vi "UHR-Fleezers Control (host) - Lorentz v3.vi"() -> ()   [LabVIEW 2014] (continued)
    n3456 = Bundle By Name(cluster=w4564, "Set 1"=w4563, "Set 2"=w4562) -> (w4334:cluster{"Set 1":dbl, "Set 2":dbl})
    n3457 = Divide(x=w4447, y=327.67) -> (x/y=→"Action (%)":dbl)
    n3458 = case shown="True" "Semi Passive Mode" {
      tunnel: w4313 -> [_ w4631]
      frame False {
      }
      frame True {
        n3459 = local read "Target Force (pN)"() -> (w4629:dbl)
        n3460 = Less?(x="Jump Force (pN)", y=w4629) -> (x < y?=w4627:bool)
        n3461 = case shown="False" w4627 {
          tunnel: "Jump Force (pN)" -> [w4637 w4640]
          tunnel: w4631 -> [w4636 w4639]
          tunnel: [w4635 w4638] -> w4630
          frame False {
            n3462 = Less?(x=w4637, y=w4636) -> (x < y?=w4635:bool)
          }
          frame True {
            n3463 = Greater?(x=w4640, y=w4639) -> (0:w4638:bool)
          }
        }
        n3464 = case shown="False" w4630 {
          frame False {
            n3465 = local read "Trap Pos. FB ON"() -> (w4632:bool)
            n3466 = case shown="False" w4632 {
              frame False {
              }
              frame True {
                n3467 = property on="Trap Pos. FB ON" class="Bool (strict)"("Val(Sgnl)"=FALSE) -> ()  [unwired: 2 in, 2 out]
              }
            }
          }
          frame True {
            n3468 = property on="Trap Pos. FB ON" class="Bool (strict)"("Val(Sgnl)"=TRUE) -> ()  [unwired: 2 in, 2 out]
          }
        }
      }
    }
    n3469 = local read "Trap X (AI1)"() -> (w4467:T15)
    n3470 = call "IR AOM word double to freq.vi"("Frequency Word In (double)"=w4405) -> ("Frequency Out (MHz)"=w4404:dbl)
    n3471 = call "IR AOM word double to freq.vi"("Frequency Word In (double)"=w4407) -> ("Frequency Out (MHz)"=w4406:dbl)
    n3472 = Divide(x=w4334, y=3276.7) -> (x/y=w4560:cluster{"Set 1":dbl, "Set 2":dbl})
    n3473 = Multiply(x=w4406, y=w4413) -> (x*y=w4412:dbl)
    "TTrig Sig (nm)" <- w4412
    n3474 = Multiply(x=w4404, y=w4413) -> (x*y=w4411:dbl)
    "TTrig Fin Thresh (nm)" <- w4411
    n3475 = local write "AI2 (V)"(w4560) -> ()
    n3476 = Bundle(cluster=w4467, "Trap 1"=w4454, "Trap 2"=w4453) -> (→"Trap X (AI1)":T15)
    n3477 = local read "Trap Pos. FB ON"() -> (w4320:bool)
    n3478 = local read "Dynamic Force FB (ronen)"() -> (w4321:bool)
    n3479 = Bundle(w4412, w4411) -> (→"TTrig":cluster{dbl, dbl})  [unwired: 1 in]
    n3480 = Compound Arithmetic op=AND(w4321, "Real time Offset file correction for setpoint", w4320) -> (w4322:bool)
    n3481 = case shown="True" w4322 {
      tunnel: w4332 -> [_ _]
      tunnel: w4318 -> [_ w4659]
      tunnel: w4315 -> [_ w4642]
      frame False {
      }
      frame True {
        # "Changed by Ronen - real time update of set point\naccording to offset file"
        n3482 = local read "T1 calibration"() -> (w4654:T9)
        n3483 = local read "Offset file step size"() -> (w4661:dbl)
        n3484 = local read "Setpoint offset\ncorrection values"() -> (w4658:dbl[])
        n3485 = Multiply(x="Target Force (pN)", y=2.0) -> (x*y=w4655:dbl)
        n3486 = local read "Negate Diff?"() -> (w4643:bool)
        n3487 = Unbundle By Name(w4654) -> ("T1 alpha_x (nm/V)"=w4653:dbl, "T1 kappa_x (pN/nm)"=w4652:dbl)
        n3488 = Divide(x=w4659, y=w4661) -> (x/y=w4662:dbl)
        n3489 = To Long Integer(number=w4662) -> (32bit integer=w4660:i32)
        n3490 = Index Array(array=w4658, index=w4660) -> (element=w4645:dbl)
        n3491 = Multiply(x=w4653, y=w4652) -> (x*y=w4651:dbl)
        n3492 = Select(t=1, s=w4643, f=-1) -> (s? t:f=w4646:i32)
        n3493 = Divide(x=w4655, y=w4651) -> (x/y=w4650:dbl)
        n3494 = Multiply(x=w4646, y=w4645) -> (x*y=w4644:dbl)
        n3495 = Add(x=w4650, y=w4644) -> (x+y=w4649:dbl)
        n3496 = To Fixed-Point(number=w4649) -> (fixed-point=w4641:fxp<+/-,16,1>)  [unwired: 1 in]
        "Actual Setpoint" <- w4641
        n3497 = xnode "Read/Write Control"("FPGA VI Reference In"=w4642, "Trap Pos. FB SP"=w4641) -> ()  [unwired: 1 in, 2 out]
      }
    }
    n3498 = local read "All FB On/Off"() -> (w4333:bool)
    n3499 = case shown="True" w4333 {
      tunnel: w4334 -> [_ w4665]
      frame False {
      }
      frame True {
        n3500 = Divide(x=w4665, y=3276.7) -> (x/y=w4663:cluster{"Set 1":dbl, "Set 2":dbl})
        n3501 = Unbundle By Name(w4663) -> ("Set 1"=w4670:dbl, "Set 2"=w4669:dbl)
        n3502 = Greater?(x=w4670, y="Feedback Auto-Off threshold") -> (0:w4668:bool)
        n3503 = Greater?(x=w4669, y="Feedback Auto-Off threshold") -> (0:w4667:bool)
        n3504 = Or(x=w4668, y=w4667) -> (x .or. y?=w4666:bool)
        n3505 = case shown="True" w4666 {
          frame False {
          }
          frame True {
            n3506 = property on="All FB On/Off" class="Bool (strict)"("Val(Sgnl)"=FALSE) -> ()  [unwired: 2 in, 2 out]
          }
        }
      }
    }
    n3507 = flat-sequence "To save data" {
      tunnel: [w5368] -> w4583
      tunnel: [w5369] -> w4582
      tunnel: w4545 -> [w5362]
      tunnel: w4256 -> [w5366]
      tunnel: ["Save Calibration"] -> w4557
      tunnel: w4304 -> [w5365]
      tunnel: [w5358] -> w4554
      tunnel: [w5355] -> w4553
      tunnel: [w5352] -> w4552
      tunnel: w4544 -> [w5354]
      tunnel: w4283 -> [w5348]
      tunnel: [w5348] -> w4508
      tunnel: ["Start Saving"] -> w4488
      tunnel: [w5343] -> w4437
      tunnel: [w5342] -> w4436
      tunnel: [w5339] -> w4338
      tunnel: [w5335] -> w4326
      tunnel: w4583 -> [w5680]
      tunnel: w4582 -> [w5679]
      tunnel: w4305 -> [w5678]
      tunnel: w4557 -> [w5677]
      tunnel: w4554 -> [w5675]
      tunnel: w4553 -> [w5674]
      tunnel: w4552 -> [w5673]
      tunnel: w4279 -> [w5672]
      tunnel: w4300 -> [w5671]
      tunnel: w4508 -> [w5670]
      tunnel: w4488 -> [w5669]
      tunnel: w4345 -> [w5668]
      tunnel: w4387 -> [w5667]
      tunnel: w4437 -> [w5666]
      tunnel: w4436 -> [w5665]
      tunnel: w4435 -> [w5664]
      tunnel: w4228 -> [w5663]
      tunnel: w4294 -> [w5662]
      tunnel: w4338 -> [w5661]
      tunnel: w4326 -> [w5660]
      frame #0 {
        # "Changed by Ronen - we don't have a database so we disabled this"
        n3508 = Or(x="Save N Sets", y="Start Saving") -> (x .or. y?=w5349:bool)
        n3509 = To Double Precision Float(number=w5365) -> (double precision float=w5359:dbl)
        n3510 = Build Array(w5349, "Save Calibration", w5362, w5354, "Flow Cal") -> (w5364:bool[])
        n3511 = Compound Arithmetic op=OR("Save Calibration", w5362, w5349, w5354, "Flow Cal") -> (w5367:bool)
        n3512 = Boolean Array To Number(Boolean array=w5364) -> (number=w5361:u32)
        n3513 = feedback #21(FALSE ("Save APD Data\nwith Trap Data")) -> (w5344:bool)
        n3514 = feedback #22(refnum<k0> refnum) -> (w5370:refnum<file>)
        n3515 = feedback #23(FALSE ("Save APD Data\nwith Trap Data")) -> (w5353:bool)
        n3516 = feedback #24(0) -> (w5372:i32)
        n3517 = feedback #25() -> (w5360:u32)  [unwired: 1 out]
        n3518 = feedback #26(refnum<k0> refnum) -> (w5340:refnum<file>)
        n3519 = feedback #27(refnum<k0> refnum) -> (w5346:refnum<file>)
        n3520 = feedback #28(refnum<k0> refnum) -> (w5336:refnum<file>)
        n3521 = feedback #29(refnum<k0> refnum) -> (w5356:refnum<file>)
        n3522 = case shown="True" w5367 {
          tunnel: [w5381 1] -> w5368
          tunnel: w5372 -> [w5383 _]
          tunnel: [w5382 w5415] -> w5369
          tunnel: w5370 -> [w5382 _]
          tunnel: w5366 -> [_ w5433]
          tunnel: w5359 -> [_ w5431]
          tunnel: w5361 -> [_ w5434]
          tunnel: [w5380 w5414] -> w5358
          tunnel: w5360 -> [w5380 _]
          tunnel: [w5379 w5412] -> w5355
          tunnel: w5356 -> [w5379 _]
          tunnel: [w5378 w5411] -> w5352
          tunnel: w5353 -> [w5378 _]
          tunnel: "Start Saving" -> [_ w5409]
          tunnel: w5348 -> [_ w5408]
          tunnel: [w5377 w5401] -> w5342
          tunnel: w5346 -> [w5377 _]
          tunnel: [w5376 w5400] -> w5343
          tunnel: w5344 -> [w5376 _]
          tunnel: [w5375 w5386] -> w5339
          tunnel: w5340 -> [w5375 _]
          tunnel: [w5374 w5384] -> w5335
          tunnel: w5336 -> [w5374 _]
          frame False {
            n3523 = Increment(x=w5383) -> (x+1=w5381:i32)
          }
          frame True {
            w5385 = FALSE ("Start Saving")
            w5410 = 10.0  # File Version
            w5417 = FALSE ("prepend array or string size? (T)")
            w5416 = T45."big-endian, network order" ("byte order (0:big-endian, network order)")
            # "Ronen Changed the create file - changed data folder to c:\\Data"
            # "Save trap position\ndata"
            n3524 = Array Size(array=w5408) -> (size(s)=w5407:i32)
            n3525 = To Double Precision Float(number=w5407) -> (double precision float=w5406:dbl)
            n3526 = local read "BD 1 Frequency 1 (MHz)"() -> (w5430:dbl)
            n3527 = local read "BD 2 Frequency 1 (MHz)"() -> (w5429:dbl)
            n3528 = local read "BD 1 Frequency 2 (MHz)"() -> (w5428:dbl)
            n3529 = local read "BD 2 Frequency 2 (MHz)"() -> (w5427:dbl)
            n3530 = local read "BD 1 Frequency 3 (MHz)"() -> (w5426:dbl)
            n3531 = local read "BD 2 Frequency 3 (MHz)"() -> (w5425:dbl)
            n3532 = local write "Flow Cal"(w5385) -> ()
            n3533 = local write "Save Calibration"(w5385) -> ()
            n3534 = local write "Start Saving"(w5385) -> ()
            n3535 = Build Array("Save APD Data\nwith Trap Data", "Save Trap Pos. Data") -> (w5403:bool[])
            n3536 = Boolean Array To Number(Boolean array=w5403) -> (number=w5402:u32)
            n3537 = Build Array(w5430, w5429, w5428, w5427, w5426, w5425) -> (w5424:dbl[])
            n3538 = case shown="16" w5434 {
              tunnel: w5433 -> [w5534 w5561 w5577 w5615 w5652]
              tunnel: w5406 -> [w5539 w5568 w5597 w5634 w5657]
              tunnel: w5431 -> [w5538 w5567 w5596 w5633 w5656]
              tunnel: [w5535 w5563 w5588 w5625 w5653] -> w5422
              tunnel: [w5526 "Cal sets to save" w5578 w5616 w5639] -> w5414
              tunnel: w5424 -> [w5536 w5564 w5590 w5627 w5654]
              tunnel: "Save APD Data\nwith Trap Data" -> [w5533 w5550 w5574 w5613 w5651]
              tunnel: [w5533 w5548 w5574 w5613 w5651] -> w5411
              tunnel: w5410 -> [w5529 w5557 w5572 w5611 w5647]
              tunnel: w5409 -> [w5528 _ _ _ _]
              tunnel: [w5519 w5556 w5571 w5601 w5646] -> w5400
              tunnel: "Save Trap Pos. Data" -> [w5519 w5555 w5571 w5601 w5646]
              tunnel: w5402 -> [w5518 w5554 w5570 w5600 w5645]
              frame 1, Default {
                # "timeseries"
                n3539 = case shown="True" "Profile" {
                  tunnel: [w5542 w5546] -> w5523
                  tunnel: [w5542 w5545] -> w5522
                  tunnel: [w5542 w5544] -> w5521
                  tunnel: [w5542 w5543] -> w5520
                  frame False {
                    w5542 = 0.0 ("f")
                  }
                  frame True {
                    n3540 = local read "Current Position"() -> (w5547:cluster{dbl, dbl, dbl})
                    n3541 = local read "Y change (mm)"() -> (w5543:dbl)
                    n3542 = Unbundle(w5547) -> (w5546:dbl, w5545:dbl, w5544:dbl)
                  }
                }
                n3543 = local read "Save ave N"() -> (w5541:dbl)
                n3544 = Multiply(x=w5541, y=w5534) -> (x*y=w5540:dbl)
                n3545 = To Double Precision Float(number=w5518) -> (double precision float=w5532:dbl)
                n3546 = Build Array(w5529, w5534, w5540, w5539, w5538, 0.0 ("f")) -> (w5537:dbl[])
                n3547 = Build Array(w5532, w5523, w5522, w5521, w5520) -> (w5530:dbl[])
                n3548 = Select(t=u32 4000000000, s=w5528, f="N sets to save") -> (s? t:f=w5526:u32)
                n3549 = Build Array (concatenate)(w5537, w5536, w5530) -> (w5535:dbl[])
              }
              frame 2 {
                w5559 = 0.0 ("f")
                w5549 = FALSE ("Save APD Data\nwith Trap Data")
                # "For diagnostics save trap position\ndata during cal"
                # "calibration"
                n3550 = Boolean To (0,1)(Boolean=w5549) -> (0, 1=w5553:i16)
                n3551 = Select(t=w5550, s="Save trap pos with cal", f=w5549) -> (s? t:f=w5548:bool)
                n3552 = Select(t=w5555, s="Save trap pos with cal", f=w5549) -> (s? t:f=w5556:bool)
                n3553 = Select(t=w5554, s="Save trap pos with cal", f=w5553) -> (s? t:f=w5552:u32)
                n3554 = To Double Precision Float(number=w5552) -> (double precision float=w5560:dbl)
                n3555 = Build Array(w5557, w5561, w5561, w5568, w5567, 1.0 ("t")) -> (w5565:dbl[])
                n3556 = Build Array(w5560, w5559, w5559, w5559, w5559) -> (w5558:dbl[])
                n3557 = Build Array (concatenate)(w5565, w5564, w5558) -> (w5563:dbl[])
                "Calibrating Trap..." <- TRUE ("Calibrating...")
              }
              frame 4 {
                w5575 = 0.0 ("f")
                # "scan dir (x/y = 0/1)"
                # "cycles/step"
                # "n scans (f/b)"
                # "steps"
                # "freq. range"
                # "AOD raster scan"
                n3558 = local read "Number of F/B Scans (AOD)"() -> (w5582:u16)
                n3559 = local read "Cycles/step (AOD)"() -> (w5584:u64)
                n3560 = local read "Scan Range (MHz)"() -> (w5587:dbl)
                n3561 = local read "Scan steps (AOD)"() -> (w5586:u64)
                n3562 = local read "Scan BD"() -> (w5594:bool)
                n3563 = local read "Save ave N"() -> (w5599:dbl)
                n3564 = Boolean To (0,1)(Boolean=w5594) -> (0, 1=w5593:i16)
                n3565 = To Double Precision Float(number=w5582) -> (double precision float=w5581:dbl)
                n3566 = To Double Precision Float(number=w5586) -> (double precision float=w5585:dbl)
                n3567 = To Double Precision Float(number=w5584) -> (double precision float=w5583:dbl)
                n3568 = To Double Precision Float(number=w5593) -> (double precision float=w5592:dbl)
                n3569 = Multiply(x=w5599, y=w5577) -> (x*y=w5598:dbl)
                n3570 = To Double Precision Float(number=w5570) -> (double precision float=w5576:dbl)
                n3571 = Build Array(w5576, w5575, w5575, w5575, w5575) -> (w5573:dbl[])
                n3572 = local read "N sets should be saved"() -> (w5579:dbl)
                n3573 = Build Array(w5592, w5587, w5585, w5583, w5581) -> (w5589:dbl[])
                n3574 = Build Array(w5572, w5577, w5598, w5597, w5596, 2.0 ("t")) -> (w5591:dbl[])
                n3575 = Round Toward +Infinity(x=w5579) -> (ceil(x): smallest int >= x=w5580:dbl)
                n3576 = Build Array (concatenate)(w5591, w5590, w5573, w5589) -> (w5588:dbl[])
                n3577 = To Unsigned Long Integer(number=w5580) -> (unsigned 32bit integer=w5578:u32)
              }
              frame 8 {
                w5608 = 0.0 ("f")
                # "MCL raster scan"
                n3578 = local read "Number of scans (MCL)"() -> (w5603:u64)
                n3579 = local read "2D or 1D Scan"() -> (w5605:bool)
                n3580 = local read "Scan lines (y)"() -> (w5602:u64)
                n3581 = local read "Scan Range (V)\n(of steps)"() -> (w5624:dbl)
                n3582 = local read "Fast Scan Dir"() -> (w5631:bool)
                n3583 = local read "Cycles/step (MCL)"() -> (w5621:u64)
                n3584 = local read "Scan steps (MCL)"() -> (w5623:u64)
                n3585 = Select(t=w5602, s=w5605, f=w5603) -> (s? t:f=w5604:u64)
                n3586 = Boolean To (0,1)(Boolean=w5605) -> (0, 1=w5607:i16)
                n3587 = local read "Save ave N"() -> (w5636:dbl)
                n3588 = local read "Initial X"() -> (w5610:dbl)
                n3589 = local read "Initial Y"() -> (w5609:dbl)
                n3590 = To Double Precision Float(number=w5607) -> (double precision float=w5606:dbl)
                n3591 = Boolean To (0,1)(Boolean=w5631) -> (0, 1=w5630:i16)
                n3592 = To Double Precision Float(number=w5604) -> (double precision float=w5619:dbl)
                n3593 = To Double Precision Float(number=w5623) -> (double precision float=w5622:dbl)
                n3594 = To Double Precision Float(number=w5621) -> (double precision float=w5620:dbl)
                n3595 = To Double Precision Float(number=w5630) -> (double precision float=w5629:dbl)
                n3596 = Multiply(x=w5636, y=w5615) -> (x*y=w5635:dbl)
                n3597 = To Double Precision Float(number=w5600) -> (double precision float=w5614:dbl)
                n3598 = local read "N sets should be saved (MCL)"() -> (w5617:dbl)
                n3599 = Build Array(w5614, w5606, w5608, w5608, w5608) -> (w5612:dbl[])
                n3600 = Build Array(w5629, w5624, w5622, w5620, w5619, w5610, w5609) -> (w5626:dbl[])
                n3601 = Build Array(w5611, w5615, w5635, w5634, w5633, 3.0 ("t")) -> (w5628:dbl[])
                n3602 = Round Toward +Infinity(x=w5617) -> (ceil(x): smallest int >= x=w5618:dbl)
                n3603 = Build Array (concatenate)(w5628, w5627, w5612, w5626) -> (w5625:dbl[])
                n3604 = To Unsigned Long Integer(number=w5618) -> (unsigned 32bit integer=w5616:u32)
              }
              frame 16 {
                w5638 = 0.0
                # "Flow calibration - added by Ronen: Number\nof saved sets is distance (1 mm) divided by \nspeed +1.5 spare second divided by the time of\nset measurement, 0.2 sec for 2 set interlace"
                # "timeseries"
                n3605 = local read "Save ave N"() -> (w5659:dbl)
                n3606 = Reciprocal(x=0.0) -> (1/x=w5644:dbl)
                n3607 = Add(x=w5644, y=1.5) -> (x+y=w5642:dbl)
                n3608 = Multiply(x=w5659, y=w5652) -> (x*y=w5658:dbl)
                n3609 = Divide(x=w5642, y=0.2) -> (x/y=w5640:dbl)
                n3610 = To Double Precision Float(number=w5645) -> (double precision float=w5650:dbl)
                n3611 = To Unsigned Long Integer(number=w5640) -> (unsigned 32bit integer=w5639:u32)
                n3612 = Build Array(w5647, w5652, w5658, w5657, w5656, 4.0 ("f")) -> (w5655:dbl[])
                n3613 = Build Array(w5650, w5638, w5638, w5638, w5638) -> (w5648:dbl[])
                n3614 = Build Array (concatenate)(w5655, w5654, w5648) -> (w5653:dbl[])
              }
            }
            n3615 = local read "Index"() -> (w5439:dbl)
            n3616 = call "Create new save file.vi"("Insert"="", "Ext"=".dat", "Index In"=w5439) -> ("Path Out"=w5388:path, "Index Out"=w5413:dbl)
            n3617 = local write "Save file name"(w5388) -> ()
            n3618 = local write "Index"(w5413) -> ()
            n3619 = local write "Save index"(w5413) -> ()
            n3620 = case shown="True" "Save Event Log?" {
              tunnel: w5388 -> [_ w5453]
              tunnel: [refnum<k0> refnum w5452] -> w5386
              frame False {
              }
              frame True {
                (unwired) FALSE ("prepend array or string size? (T)")
                n3621 = Path To String(path=w5453) -> (string=w5464:string)
                n3622 = String Length(string=w5464) -> (length=w5463:i32)
                n3623 = Subtract(x=w5463, y=4) -> (x-y=w5461:i32)
                n3624 = String Subset(string=w5464, length (rest)=w5461) -> (substring=w5460:string)  [unwired: 1 out]
                n3625 = Concatenate Strings(w5460, "_log.txt" ("string")) -> (w5458:string)
                n3626 = String To Path(string=w5458) -> (path=w5454:path)
                n3627 = Open/Create/Replace File(file path (use dialog)=w5454, operation (0:open)=T44."create", access (0:read/write)=enum16{"read/write", "read-only", "write-only"}."write-only") -> (refnum out=w5455:refnum<file>)  [unwired: 1 in, 4 out]
                n3628 = Deny Access(7:w5455) -> (3:w5452:refnum<file>)  [unwired: 1 in, 2 out]
                n3629 = call "write to event log.vi"("log file ref"=w5452, "time"=0.0, "input string"="start log") -> ()  [unwired: 8 in]
              }
            }
            "log file ref" <- w5386
            n3630 = Array Size(array=w5422) -> (size(s)=w5423:i32)
            n3631 = Open/Create/Replace File(file path (use dialog)=w5388, operation (0:open)=T44."create", access (0:read/write)=enum16{"read/write", "read-only", "write-only"}."write-only") -> (refnum out=w5436:refnum<file>)  [unwired: 1 in, 4 out]
            n3632 = local write "Saving..."(TRUE ("Saving...")) -> ()
            n3633 = To Double Precision Float(number=w5423) -> (double precision float=w5421:dbl)
            n3634 = String Length(string="Comment (data description)") -> (length=w5420:i32)
            n3635 = To Double Precision Float(number=w5420) -> (double precision float=w5419:dbl)
            n3636 = Deny Access(7:w5436) -> (3:w5435:refnum<file>)  [unwired: 1 in, 2 out]
            n3637 = Build Array (concatenate)(w5421, w5422, w5419) -> (w5398:dbl[])
            n3638 = case "If fluorescence data to be saved" shown="True" w5411 {
              tunnel: w5388 -> [_ w5517]
              tunnel: [w5487 w5500] -> w5412
              tunnel: [w5487 w5488] -> w5384
              frame False {
                w5487 = refnum<k0> refnum
              }
              frame True {
                w5499 = 0.0
                w5492 = T44."create" ("operation (0:open)")
                w5493 = enum16{"read/write", "read-only", "write-only"}."write-only" ("access (0:read/write)")
                n3639 = local read "APD Integration Time (s)"() -> (w5505:dbl)
                n3640 = local read "N APD Samp/step"() -> (w5498:dbl)
                n3641 = local read "Number of APDs"() -> (w5497:u8)
                n3642 = Path To String(path=w5517) -> (string=w5516:string)
                n3643 = String Length(string=w5516) -> (length=w5515:i32)
                n3644 = Subtract(x=w5515, y=4) -> (x-y=w5513:i32)
                n3645 = String Subset(string=w5516, length (rest)=w5513) -> (substring=w5496:string)  [unwired: 1 out]
                n3646 = Build Array(w5505, w5498, w5497, w5499, w5499, w5499, w5499, w5499) -> (w5502:dbl[])
                n3647 = Concatenate Strings(w5496, "_green.dat") -> (w5494:string)
                n3648 = Concatenate Strings(w5496, "_fl.dat" ("string")) -> (w5511:string)
                n3649 = Array Size(array=w5502) -> (size(s)=w5504:i32)
                n3650 = String To Path(string=w5511) -> (path=w5509:path)
                n3651 = Open/Create/Replace File(file path (use dialog)=w5509, operation (0:open)=w5492, access (0:read/write)=w5493) -> (refnum out=w5510:refnum<file>)  [unwired: 1 in, 4 out]
                n3652 = Deny Access(7:w5510) -> (3:w5506:refnum<file>)  [unwired: 1 in, 2 out]
                n3653 = String To Path(string=w5494) -> (path=w5491:path)
                n3654 = To Double Precision Float(number=w5504) -> (double precision float=w5503:dbl)
                n3655 = Build Array (concatenate)(w5503, w5502) -> (w5501:dbl[])
                n3656 = Write to Binary File(file (use dialog)=w5506, data=w5501, 5:FALSE ("prepend array or string size? (T)"), 9:T45."big-endian, network order" ("byte order (0:big-endian, network order)")) -> (refnum out=w5500:refnum<file>)  [unwired: 1 in, 3 out]
                n3657 = Open/Create/Replace File(file path (use dialog)=w5491, operation (0:open)=w5492, access (0:read/write)=w5493) -> (refnum out=w5489:refnum<file>, error out=w5490:errorcluster)  [unwired: 3 in, 1 out]
                n3658 = Deny Access(4:w5490, 7:w5489) -> (3:w5488:refnum<file>)  [unwired: 1 in, 1 out]
              }
            }
            n3659 = case shown="True" w5400 {
              tunnel: w5388 -> [_ w5472]
              tunnel: [refnum<k0> refnum w5471] -> w5401
              frame False {
              }
              frame True {
                w5467 = 0.0 ("element")
                n3660 = Path To String(path=w5472) -> (string=w5486:string)
                n3661 = Build Array(w5467, w5467, w5467, w5467, w5467, w5467, w5467, w5467) -> (w5468:dbl[])
                n3662 = String Length(string=w5486) -> (length=w5485:i32)
                n3663 = Subtract(x=w5485, y=4) -> (x-y=w5483:i32)
                n3664 = Array Size(array=w5468) -> (size(s)=w5470:i32)
                n3665 = String Subset(string=w5486, length (rest)=w5483) -> (substring=w5482:string)  [unwired: 1 out]
                n3666 = To Double Precision Float(number=w5470) -> (double precision float=w5469:dbl)
                n3667 = Concatenate Strings(w5482, "_pos.dat" ("string")) -> (w5480:string)
                n3668 = Build Array (concatenate)(w5469, w5468) -> (w5466:dbl[])
                n3669 = String To Path(string=w5480) -> (path=w5476:path)
                n3670 = Open/Create/Replace File(file path (use dialog)=w5476, operation (0:open)=T44."create", access (0:read/write)=enum16{"read/write", "read-only", "write-only"}."write-only") -> (refnum out=w5477:refnum<file>)  [unwired: 1 in, 4 out]
                n3671 = Deny Access(7:w5477) -> (3:w5473:refnum<file>)  [unwired: 1 in, 2 out]
                n3672 = Write to Binary File(file (use dialog)=w5473, data=w5466, 5:FALSE ("prepend array or string size? (T)"), 9:T45."big-endian, network order" ("byte order (0:big-endian, network order)")) -> (refnum out=w5471:refnum<file>)  [unwired: 1 in, 3 out]
              }
            }
            n3673 = Write to Binary File(file (use dialog)=w5435, data=w5398, 5:w5417, 9:w5416) -> (refnum out=w5418:refnum<file>)  [unwired: 1 in, 3 out]
            n3674 = Write to Binary File(file (use dialog)=w5418, data="Comment (data description)", 5:w5417, 9:w5416) -> (refnum out=w5415:refnum<file>)  [unwired: 1 in, 3 out]
            n3675 = local read "connection reference"() -> (w5399:T25)
            n3676 = Bundle("Comment (data description)"="Comment (data description)", "Channel 1 Buffer"="Channel 1 Buffer", "Channel 2 Buffer"="Channel 2 Buffer", "Channel 3 Buffer"="Channel 3 Buffer", "Title"="Title", "DNA Construct"="DNA Construct", "Bead diameter"="Bead diameter", "Name"="Name") -> (w5389:T64)  [unwired: 1 in]
            n3677 = disable-structure shown="Disabled" {
              disable-tunnel: w5399 -> [w5447 _]
              disable-tunnel: w5398 -> [w5445 _]
              disable-tunnel: w5389 -> [w5444 _]
              disable-tunnel: w5388 -> [w5443 _]
              frame Disabled {
                n3678 = call "MattFileCreator-v9.vi"("Comments"=w5444, "Input Array"=w5445, "File path"=w5443, "table"="labview", "connection reference"=w5447) -> ("connection reference out"=w5446:T25)  [unwired: 5 in, 1 out]
                n3679 = local write "connection reference"(w5446) -> ()
              }
              frame Enabled {
              }
            }
          }
        }
        n3680 = feedback-in #21(w5343) -> ()
        n3681 = feedback-in #22(w5369) -> ()
        n3682 = feedback-in #23(w5352) -> ()
        n3683 = feedback-in #24(w5368) -> ()
        n3684 = feedback-in #25(w5358) -> ()
        n3685 = feedback-in #26(w5339) -> ()
        n3686 = feedback-in #27(w5342) -> ()
        n3687 = feedback-in #28(w5335) -> ()
        n3688 = feedback-in #29(w5355) -> ()
      }
      frame #1 {
        n3689 = local read "Saving..."() -> (w5676:bool)
        n3690 = case shown="True" w5676 {
          tunnel: w5680 -> [_ w5694]
          tunnel: w5679 -> [_ w5708]
          tunnel: w5678 -> [_ w5704]
          tunnel: w5677 -> [_ w5703]
          tunnel: w5675 -> [_ w5702]
          tunnel: w5674 -> [_ w5697]
          tunnel: w5673 -> [_ w5696]
          tunnel: w5672 -> [_ w5695]
          tunnel: w5671 -> [_ w5693]
          tunnel: w5670 -> [_ w5691]
          tunnel: w5669 -> [_ w5690]
          tunnel: w5668 -> [_ w5689]
          tunnel: w5667 -> [_ w5688]
          tunnel: w5666 -> [_ w5687]
          tunnel: w5665 -> [_ w5686]
          tunnel: w5664 -> [_ w5685]
          tunnel: w5663 -> [_ w5684]
          tunnel: w5662 -> [_ w5683]
          tunnel: w5661 -> [_ w5682]
          tunnel: w5660 -> [_ w5681]
          frame False {
          }
          frame True {
            n3691 = Multiply(x=w5694, y=w5693) -> (x*y=→"Time (s)":dbl)
            n3692 = Less Or Equal?(x=w5694, y=w5702) -> (x <= y?=w5706:bool)
            n3693 = Compound Arithmetic op=OR("Stop Saving", "Abort save 2") -> (w5698:bool)
            n3694 = Not(x=w5698) -> (.not. x?=w5707:bool)
            n3695 = And(x=w5706, y=w5707) -> (x .and. y?=w5705:bool)
            n3696 = case shown="True" w5705 {
              tunnel: w5708 -> [w5718 w5819]
              tunnel: [0.0 w5822] -> w5701
              tunnel: w5694 -> [_ w5820]
              tunnel: w5702 -> [_ w5821]
              tunnel: w5704 -> [_ w5816]
              tunnel: w5703 -> [_ _]
              tunnel: w5697 -> [w5716 w5809]
              tunnel: w5696 -> [w5715 w5810]
              tunnel: w5695 -> [_ w5808]
              tunnel: w5691 -> [_ w5807]
              tunnel: w5690 -> [_ w5725]
              tunnel: w5689 -> [_ w5800]
              tunnel: w5688 -> [_ w5747]
              tunnel: w5687 -> [w5712 w5764]
              tunnel: w5686 -> [w5713 w5763]
              tunnel: w5685 -> [_ w5760]
              tunnel: w5684 -> [_ w5758]
              tunnel: w5683 -> [_ w5724]
              tunnel: w5682 -> [w5711 _]
              tunnel: w5681 -> [w5709 w5723]
              frame False {
                w5714 = FALSE
                n3697 = Close File(refnum=w5718) -> ()  [unwired: 1 in, 2 out]
                n3698 = case shown="True" w5715 {
                  tunnel: w5716 -> [_ w5722]
                  tunnel: w5709 -> [_ w5721]
                  frame False {
                  }
                  frame True {
                    n3699 = Close File(refnum=w5722) -> ()  [unwired: 1 in, 2 out]
                    n3700 = Close File(refnum=w5721) -> ()  [unwired: 1 in, 2 out]
                  }
                }
                n3701 = case shown="True" w5712 {
                  tunnel: w5713 -> [_ w5720]
                  frame False {
                  }
                  frame True {
                    n3702 = Close File(refnum=w5720) -> ()  [unwired: 1 in, 2 out]
                  }
                }
                n3703 = local read "Save Event Log?"() -> (w5710:bool)
                n3704 = case shown="True" w5710 {
                  tunnel: w5711 -> [_ w5719]
                  frame False {
                  }
                  frame True {
                    n3705 = Close File(refnum=w5719) -> ()  [unwired: 1 in, 2 out]
                  }
                }
                n3706 = local write "Raster Scanning..."(w5714) -> ()
                n3707 = local write "Calibrating Trap..."(w5714) -> ()
                n3708 = call <vilib>:"Beep.vi"() -> ()  [unwired: 3 in, 9 out]
                n3709 = local write "Stop Saving"(w5714) -> ()
                "Saving..." <- w5714
              }
              frame True {
                n3710 = local read "Calibrating Trap..."() -> (w5811:bool)
                n3711 = case "Write fl. data" shown="True" w5810 {
                  tunnel: w5809 -> [_ w5852]
                  tunnel: w5808 -> [_ w5851]
                  tunnel: w5723 -> [_ w5845]
                  frame False {
                  }
                  frame True {
                    w5844 = FALSE ("prepend array or string size? (T)")
                    w5846 = T45."big-endian, network order" ("byte order (0:big-endian, network order)")
                    n3712 = property on="Green Laser ON" class="Bool (strict)"() -> ("Value"=w5850:bool)  [unwired: 2 in, 2 out]
                    n3713 = property on="Green Intensity % (FB OFF)" class="DigNum (strict)"() -> ("Value"=w5849:dbl)  [unwired: 2 in, 2 out]
                    n3714 = Boolean To (0,1)(Boolean=w5850) -> (0, 1=w5848:i16)
                    n3715 = Multiply(x=w5848, y=w5849) -> (x*y=w5847:dbl)
                    n3716 = Write to Binary File(file (use dialog)=w5852, data=w5851, 5:w5844, 9:w5846) -> ()  [unwired: 1 in, 4 out]
                    n3717 = Write to Binary File(file (use dialog)=w5845, data=w5847, 5:w5844, 9:w5846) -> ()  [unwired: 2 in, 3 out]
                  }
                }
                n3718 = Greater?(x="Save ave N", y=1.0) -> (0:w5814:bool)
                n3719 = Not(x=w5811) -> (.not. x?=w5813:bool)
                n3720 = And(x=w5813, y=w5814) -> (x .and. y?=w5761:bool)
                n3721 = case shown="True" w5761 {
                  tunnel: w5760 -> [w5825 w5836]
                  tunnel: [w5825 w5828] -> w5759
                  tunnel: "Save ave N" -> [_ w5829]
                  frame False {
                  }
                  frame True {
                    w5826 = 2 ("dimension size")
                    n3722 = Array Size(array=w5836) -> (size(s)=w5830:i32)
                    n3723 = Divide(x=w5830, y=w5826) -> (x/y=w5834:dbl)
                    n3724 = Reshape Array(w5836, w5834, w5826) -> (w5835:u64[][])
                    n3725 = Transpose 2D Array(2D array=w5835) -> (transposed array=w5833:u64[][])
                    n3726 = for {
                      tunnel: w5833 -> [w5838] mode=indexing
                      tunnel: [w5837] -> w5827 mode=indexing
                      tunnel: w5829 -> [w5839]
                      workers-P: _ -> [_]
                      n3727 = call "downsample 1D array - U64.vi"("Ave N"=w5839, "Array In"=w5838) -> ("Array Out"=w5837:u64[])  [unwired: 1 in]
                    }
                    n3728 = Transpose 2D Array(2D array=w5827) -> (transposed array=w5832:u64[][])
                    n3729 = Divide(x=w5830, y=w5829) -> (x/y=w5831:dbl)
                    n3730 = Reshape Array(w5832, w5831) -> (w5828:u64[])
                  }
                }
                n3731 = case shown="True" w5761 {
                  tunnel: w5816 -> [w5853 w5865]
                  tunnel: [w5853 w5857] -> w5812
                  tunnel: "Save ave N" -> [_ w5858]
                  tunnel: w5807 -> [_ w5856]
                  frame False {
                  }
                  frame True {
                    n3732 = Array Size(array=w5865) -> (size(s)=w5859:i32)
                    n3733 = Array Size(array=w5856) -> (size(s)=w5855:i32)
                    n3734 = Divide(x=w5859, y=w5855) -> (x/y=w5863:dbl)
                    n3735 = Reshape Array(w5865, w5863, w5855) -> (w5864:i16[][])
                    n3736 = Transpose 2D Array(2D array=w5864) -> (transposed array=w5862:i16[][])
                    n3737 = for {
                      tunnel: w5862 -> [w5868] mode=indexing
                      tunnel: [w5867] -> w5854 mode=indexing
                      tunnel: w5858 -> [w5866]
                      workers-P: _ -> [_]
                      n3738 = call "downsample 1D array - I16 to F32.vi"("Ave N"=w5866, "Array In"=w5868) -> ("Array Out"=w5867:sgl[])  [unwired: 1 in]
                    }
                    n3739 = Transpose 2D Array(2D array=w5854) -> (transposed array=w5861:sgl[][])
                    n3740 = Divide(x=w5859, y=w5858) -> (x/y=w5860:dbl)
                    n3741 = Reshape Array(w5861, w5860) -> (w5857:sgl[])
                  }
                }
                n3742 = Index Array(array=w5747, index=2) -> (element=w5748:waveform(dbl))
                n3743 = Index Array(array=w5747, index=1) -> (element=w5781:waveform(dbl))
                n3744 = Index Array(array=w5747, index=0) -> (element=w5783:waveform(dbl))
                n3745 = Unbundle By Name(w5748) -> ("Y"=w5750:dbl[])
                n3746 = Unbundle By Name(w5781) -> ("Y"=w5785:dbl[])
                n3747 = Unbundle By Name(w5783) -> ("Y"=w5793:dbl[])
                n3748 = case "Write trap pos. data" shown="True" w5764 {
                  tunnel: w5763 -> [_ w5841]
                  tunnel: w5759 -> [_ w5840]
                  frame False {
                  }
                  frame True {
                    n3749 = Write to Binary File(file (use dialog)=w5841, data=w5840, 5:FALSE ("prepend array or string size? (T)"), 9:T45."big-endian, network order" ("byte order (0:big-endian, network order)")) -> ()  [unwired: 1 in, 4 out]
                  }
                }
                n3750 = Write to Binary File(file (use dialog)=w5819, data=w5812, 5:FALSE ("prepend array or string size? (T)"), 9:T45."big-endian, network order" ("byte order (0:big-endian, network order)")) -> ()  [unwired: 1 in, 4 out]
                n3751 = feedback #30(w5750) -> (w5751:dbl[])
                n3752 = Build Array (concatenate)(w5751, w5750) -> (w5746:dbl[])
                n3753 = Select(t=w5750, s=w5725, f=w5746) -> (s? t:f=w5736:dbl[])
                n3754 = feedback-in #30(w5736) -> ()
                n3755 = feedback #31(w5785) -> (w5787:dbl[])
                n3756 = Build Array (concatenate)(w5787, w5785) -> (w5786:dbl[])
                n3757 = Select(t=w5785, s=w5725, f=w5786) -> (s? t:f=w5775:dbl[])
                n3758 = feedback-in #31(w5775) -> ()
                n3759 = feedback #32(w5793) -> (w5806:dbl[])
                n3760 = Build Array (concatenate)(w5806, w5793) -> (w5805:dbl[])
                n3761 = Select(t=w5793, s=w5725, f=w5805) -> (s? t:f=w5780:dbl[])
                n3762 = feedback-in #32(w5780) -> ()
                n3763 = Divide(x=w5820, y=w5821) -> (x/y=w5823:dbl)
                n3764 = Multiply(x=w5823, y=100.0) -> (x*y=w5822:dbl)
                n3765 = Build Array(w5780, w5775, w5736) -> (→"Saved APD":dbl[][])
                n3766 = Array Size(array=w5780) -> (size(s)=w5798:i32)
                n3767 = Unbundle By Name(w5800) -> ("Y"=w5804:dbl[])
                n3768 = Subtract(x=w5798, y="N pts to average") -> (x-y=w5733:i32)
                n3769 = Multiply(x="N pts to average", y=u16 2) -> (x*y=w5776:u16)
                n3770 = Subtract(x=w5798, y=w5776) -> (x-y=w5734:i32)
                n3771 = feedback #33(w5804) -> (w5803:dbl[])
                n3772 = Build Array (concatenate)(w5803, w5804) -> (w5802:dbl[])
                n3773 = Select(t=w5804, s=w5725, f=w5802) -> (s? t:f=w5801:dbl[])
                "Trap Delta Graph" <- w5801
                n3774 = feedback-in #33(w5801) -> ()
                n3775 = Array Subset(array=w5780, index=w5733, length="N pts to average") -> (w5797:dbl[])
                n3776 = Array Subset(array=w5780, index=w5734, length="N pts to average") -> (w5796:dbl[])
                n3777 = Array Subset(array=w5775, index=w5733, length="N pts to average") -> (w5778:dbl[])
                n3778 = Array Subset(array=w5775, index=w5734, length="N pts to average") -> (w5777:dbl[])
                n3779 = Array Subset(array=w5736, index=w5733, length="N pts to average") -> (w5745:dbl[])
                n3780 = Array Subset(array=w5736, index=w5734, length="N pts to average") -> (w5744:dbl[])
                n3781 = Index Array(array=w5758, index=0) -> (element=w5756:waveform(dbl))
                n3782 = call-poly <vilib>:"Mean.vi"("X"=w5797) -> ("mean"=w5795:dbl)  [unwired: 1 out]
                n3783 = call-poly <vilib>:"Mean.vi"("X"=w5778) -> ("mean"=w5774:dbl)  [unwired: 1 out]
                n3784 = call-poly <vilib>:"Mean.vi"("X"=w5796) -> ("mean"=w5794:dbl)  [unwired: 1 out]
                n3785 = call-poly <vilib>:"Mean.vi"("X"=w5777) -> ("mean"=w5773:dbl)  [unwired: 1 out]
                n3786 = call-poly <vilib>:"Mean.vi"("X"=w5745) -> ("mean"=w5743:dbl)  [unwired: 1 out]
                n3787 = call-poly <vilib>:"Mean.vi"("X"=w5744) -> ("mean"=w5742:dbl)  [unwired: 1 out]
                n3788 = Unbundle By Name(w5756) -> ("Y"=w5754:dbl[])
                n3789 = Subtract(x=w5774, y=w5773) -> (x-y=w5765:dbl)
                "Delta Fl. 2" <- w5765
                n3790 = Subtract(x=w5743, y=w5742) -> (x-y=w5737:dbl)
                "Delta Fl. 3" <- w5737
                n3791 = Subtract(x=w5795, y=w5794) -> (x-y=w5792:dbl)
                "Delta Fl. 1" <- w5792
                n3792 = feedback #34(w5754) -> (w5753:dbl[])
                n3793 = Build Array (concatenate)(w5753, w5754) -> (w5755:dbl[])
                n3794 = Initialize Array(w5792, 1 ("dimension size")) -> (w5789:dbl[])
                n3795 = Initialize Array(w5765, 1 ("dimension size")) -> (w5770:dbl[])
                n3796 = Initialize Array(w5737, 1 ("dimension size")) -> (w5739:dbl[])
                n3797 = Select(t=w5754, s=w5725, f=w5755) -> (s? t:f=w5752:dbl[])
                "Saved trap pos" <- w5752
                n3798 = feedback-in #34(w5752) -> ()
                n3799 = feedback #35(w5789) -> (w5790:dbl[])
                n3800 = Build Array (concatenate)(w5790, w5789) -> (w5788:dbl[])
                n3801 = feedback #36(w5770) -> (w5771:dbl[])
                n3802 = feedback #37(w5739) -> (w5740:dbl[])
                n3803 = Build Array (concatenate)(w5771, w5770) -> (w5769:dbl[])
                n3804 = Build Array (concatenate)(w5740, w5739) -> (w5738:dbl[])
                n3805 = Select(t=w5789, s=w5725, f=w5788) -> (s? t:f=w5768:dbl[])
                n3806 = feedback-in #35(w5768) -> ()
                n3807 = Select(t=w5770, s=w5725, f=w5769) -> (s? t:f=w5767:dbl[])
                n3808 = feedback-in #36(w5767) -> ()
                n3809 = Select(t=w5739, s=w5725, f=w5738) -> (s? t:f=w5732:dbl[])
                n3810 = feedback-in #37(w5732) -> ()
                n3811 = Build Array(w5768, w5767, w5732) -> (→"Save APD Deriv":dbl[][])
                n3812 = Index Array(array=w5724, index=15) -> (element=w5730:waveform(dbl))
                n3813 = Unbundle By Name(w5730) -> ("Y"=w5728:dbl[])
                n3814 = feedback #38(w5728) -> (w5727:dbl[])
                n3815 = Build Array (concatenate)(w5727, w5728) -> (w5729:dbl[])
                n3816 = Select(t=w5728, s=w5725, f=w5729) -> (s? t:f=w5726:dbl[])
                "Amp current" <- w5726
                n3817 = feedback-in #38(w5726) -> ()
              }
            }
            "Progress" <- w5701
            "Progress 2" <- w5701
          }
        }
      }
    }
    n3818 = local read "wait to reset values"() -> (w4567:bool)
    n3819 = Not(x=w4565) -> (.not. x?=w4568:bool)
    n3820 = And(x=w4568, y=w4567) -> (x .and. y?=w4569:bool)
    n3821 = case "Part of MCL raster scanning: returns to initial positions after scan done" shown="True" w4569 {
      tunnel: w4315 -> [w5164 w5171]
      tunnel: [w5164 w5170] -> w4571
      tunnel: w4416 -> [w5163 w5169]
      tunnel: [w5163 w5168] -> w4566
      frame False {
      }
      frame True {
        w5179 = 10.0 ("y")
        w5178 = 32767.0 ("y")
        # "to return scan values\nafter a synchronous \nAOM scan"
        n3822 = local read "AO2"() -> (w5172:dbl)
        n3823 = local read "AO1"() -> (w5173:dbl)
        n3824 = local write "wait to reset values"(FALSE ("wait to reset values")) -> ()
        n3825 = Multiply(x=w5173, y=w5178) -> (x*y=w5175:dbl)
        n3826 = Multiply(x=w5172, y=w5178) -> (x*y=w5177:dbl)
        n3827 = Divide(x=w5175, y=w5179) -> (x/y=w5174:dbl)
        n3828 = Divide(x=w5177, y=w5179) -> (x/y=w5176:dbl)
        n3829 = To Word Integer(number=w5174) -> (16bit integer=w5180:i16)
        n3830 = To Word Integer(number=w5176) -> (16bit integer=w5181:i16)
        n3831 = local read "Total Counts (ticks)"() -> (w5165:u16)
        n3832 = local read "Scan Range (V)\n(of steps)"() -> (w5166:dbl)
        n3833 = xnode "Read/Write Control"("FPGA VI Reference In"=w5171, "error in"=w5169, "AO1"=w5180, "AO2"=w5181, "MCL count"=w5165) -> ("FPGA VI Reference Out"=w5170:T36, "error out"=w5168:errorcluster)
        n3834 = property on="Scan Range (V)\n(of steps)" class="DigNum (strict)"("Val(Sgnl)"=w5166) -> ()  [unwired: 2 in, 2 out]
      }
    }
    n3835 = case shown="True" "Sound ON" {
      tunnel: [w4684 w4729] -> w4368
      tunnel: w4367 -> [w4684 w4728]
      tunnel: w4365 -> [_ _]
      tunnel: w4344 -> [_ w4687]
      tunnel: w4364 -> [_ _]
      tunnel: w4363 -> [_ w4698]
      tunnel: w4362 -> [_ w4708]
      frame False {
      }
      frame True {
        n3836 = Index Array(array=w4687, index="Data channel to sound") -> (element=w4686:waveform(dbl))
        "Waveform Graph 2" <- w4686
        n3837 = Unbundle By Name(w4686) -> ("dt"=w4712:dbl, "Y"=w4710:dbl[])
        n3838 = Array Size(array=w4710) -> (size(s)=w4711:i32)
        "N data samples" <- w4711
        n3839 = for "Data time base" {
          N: w4711 -> [_]
          tunnel: [w4733] -> w4713 mode=indexing
          i -> [w4733]
        }
        n3840 = Multiply(x=w4712, y=w4713) -> (x*y=w4709:dbl[])
        n3841 = Compound Arithmetic op=MULTIPLY(6.283185307179586, "Carrier Frequency (Hz)", w4708) -> (w4725:dbl[])
        n3842 = call <vilib>:"Interpolate 1D.vi"("X is monotonic"=TRUE, "xi"=w4708, "X"=w4709, "Y"=w4710) -> ("yi"=w4706:dbl[])  [unwired: 5 in, 2 out]
        n3843 = Sine(x=w4725) -> (sin(x)=w4714:dbl[])
        n3844 = Add(x=w4706, y="Offset") -> (x+y=w4704:dbl[])
        n3845 = Multiply(x=w4704, y="mult x") -> (x*y=w4702:dbl[])
        n3846 = Add(x="Offset 2", y=w4702) -> (x+y=w4697:dbl[])
        n3847 = Compound Arithmetic op=MULTIPLY(6.283185307179586, "Carrier Frequency (Hz)", w4698, w4697) -> (w4689:dbl[])
        n3848 = for "Cumulative sum" {
          tunnel: [w4732] -> w4695 mode=indexing
          shift-right: [w4732] -> w4692
          shift-left: 0.0 -> [w4731]
          tunnel: w4689 -> [w4730] mode=indexing
          n3849 = Add(x=w4730, y=w4731) -> (x+y=w4732:dbl)
        }
        n3850 = feedback #39(0.0) -> (w4691:dbl)
        n3851 = Add(x=w4695, y=w4691) -> (x+y=w4694:dbl[])
        n3852 = Add(x=w4692, y=w4691) -> (x+y=w4690:dbl)
        n3853 = feedback-in #39(w4690) -> ()
        n3854 = Sine(x=w4694) -> (sin(x)=w4688:dbl[])
        n3855 = Select(t=w4714, s="tone or data", f=w4688) -> (s? t:f=w4720:dbl[])
        n3856 = Multiply(x=w4720, y="Volume") -> (x*y=w4718:dbl[])
        n3857 = Initialize Array(0.0 ("element"), "N initial buffer elements") -> (w4721:dbl[])
        n3858 = Multiply(x="N initial buffer elements", y=w4698) -> (x*y=→"Initial buffer time (s)":dbl)
        n3859 = Build Array (concatenate)(w4721, w4718) -> (w4723:dbl[])
        n3860 = First Call?() -> (First Call?: T/F=w4724:bool)
        n3861 = Select(t=w4723, s=w4724, f=w4718) -> (s? t:f=w4717:dbl[])
        n3862 = call-poly <vilib>:"Sound Output Write.vi"("data"=w4717, "task ID"=w4728) -> ("task ID out"=w4729:T51)  [unwired: 8 in, 1 out]
      }
    }
    n3863 = node-c288() -> ()  [unwired: 2 out]
  }
  n3864 = VISA Close(VISA resource name=w1) -> ()  [unwired: 1 in, 1 out]
  n3865 = disable-structure shown="Disabled" {
    disable-tunnel: w19 -> [w5869 _]
    frame Disabled {
      n3866 = call <vilib>:"Sound Output Clear.vi"("task ID"=w5869) -> ()  [unwired: 10 in, 1 out]
    }
    frame Enabled {
    }
  }
  n3867 = node-c288(w62) -> ()  [unwired: 1 out]
  n3868 = node-c288(w70) -> ()  [unwired: 1 out]
  n3869 = flat-sequence {
    tunnel: w77 -> [w5873]
    tunnel: w78 -> [w5874]
    tunnel: [w5872] -> w76
    tunnel: [w5871] -> w75
    tunnel: w74 -> [_]
    tunnel: w72 -> [_]
    tunnel: w68 -> [_]
    tunnel: w76 -> [w5875]
    tunnel: w75 -> [w5876]
    frame #0 {
      w5870 = FALSE ("AI to FIFO")
      n3870 = xnode "Read/Write Control"("FPGA VI Reference In"=w5874, "error in"=w5873, "AI to FIFO"=w5870, "APD to FIFO"=w5870) -> ("FPGA VI Reference Out"=w5872:T36, "error out"=w5871:errorcluster)
    }
    frame #1 {
      n3871 = xnode "Close FPGA VI Reference"("FPGA VI Reference In"=w5875, "error in"=w5876) -> ("error out"=→"error out":errorcluster)
    }
  }
